vi "variantCtrlStepIoPointer.vi"(4 "isRequired (T)":bool=TRUE, 6 "menu (get)":enum16{"get", "set"}(ring), 7 "procElement":variant, 8 "error in":errorcluster, 9 "String Value":string, 11 "StepElement in":variant) -> (0 "error out":errorcluster, 1 "I/O Pointer out":string, 2 "isFound?":bool, 3 "stepElement out":variant)   [LabVIEW 2024]
uses:
  controls/typeStepVarients.ctl
  variantCtrlString.vi
  proc.util.validateParamExist.vi
  <vilib>/Utility/error.llb/Clear Errors.vi
  util.error.create.vi
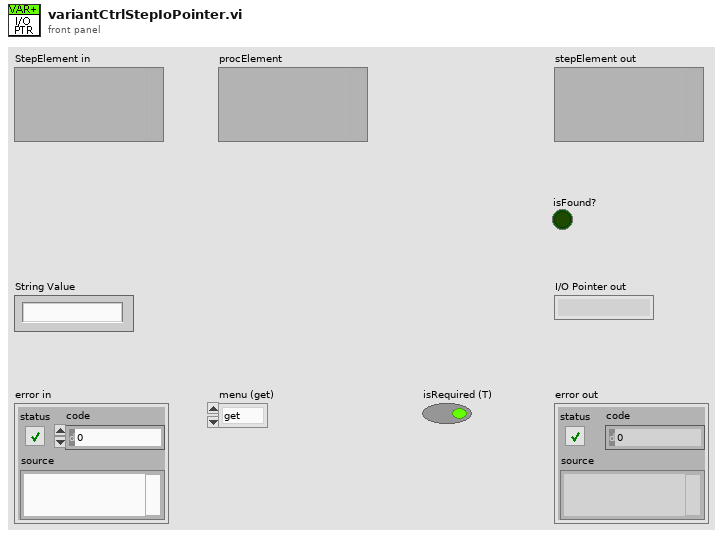
[diagram p1: front panel]
types:
  T1 = typedef "typeStepVarients.ctl" = enum16{"stepNameID", "stepFunction", "stepReport", "stepSetpoint", "stepPointer", "stepProcPointer", "stepIoPointer", "stepIoValue", "stepFilePointer", "stepMessage", "stepTimeString", "stepNumReg", "stepStrReg", "stepSeconds", "stepUnitDoseParams", "stepUnitIndex"}
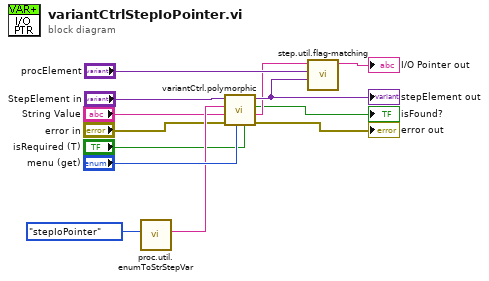
[diagram p0: block diagram]
diagram:
  n1 = call "proc.util.enumToStrStepVar.vi"("Step var"=typeStepVarients."stepIoPointer" ("proc var")) -> ("String"=w5:string)  [unwired: 10 in]
  n2 = call-poly "variantCtrl.polymorphic.vi"("isRequired (T)"="isRequired (T)", "menu in (get)"="menu (get)", "error in"="error in", "String Value"="String Value", "name in"=w5, "Step in"="StepElement in") -> ("error out"=→"error out":errorcluster, "String Value"=w8:string, "isFound?"=→"isFound?":bool, "Step out"=w12:variant)  [unwired: 2 in]
  "stepElement out" <- w12
  n3 = call "step.util.flag-matching.vi"("stepElement"=w12, "procElement"="procElement", "$string in"=w8) -> ("formated string out"=→"I/O Pointer out":string)  [unwired: 8 in]
